vi "File Write.vi"(7 "State Control":enum16{"Open", "Write", "Close"}(ring), 8 "error in (no error)":errorcluster, 10 "Event Data String":string, 11 "Event String":string) -> (0 "error out":errorcluster)   [LabVIEW 2020]
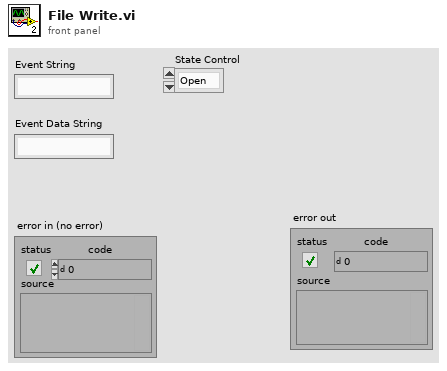
[diagram p1: front panel]
types:
  T1 = enum16{"open", "replace", "create", "open or create", "replace or create", "replace or create with confirmation"}
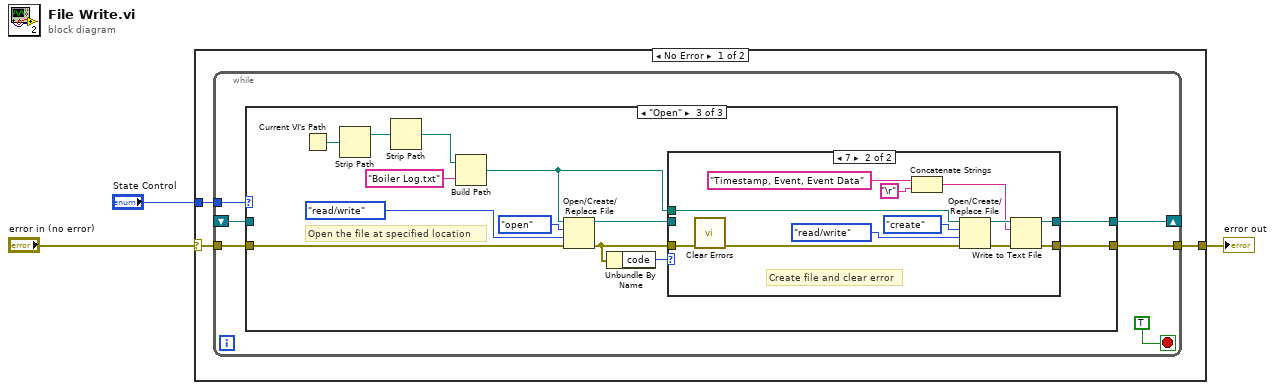
[diagram p0: block diagram]
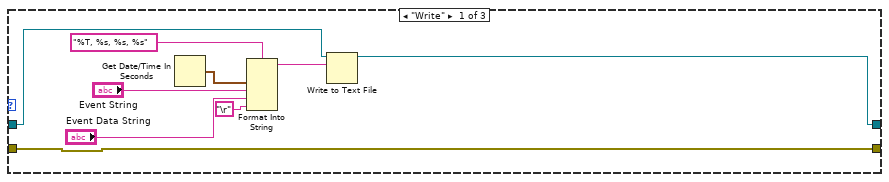
[diagram p2: hidden frame]
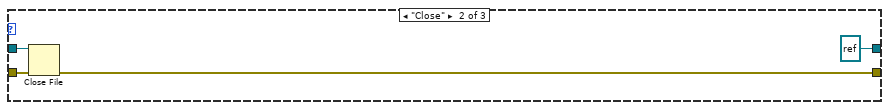
[diagram p3: hidden frame]
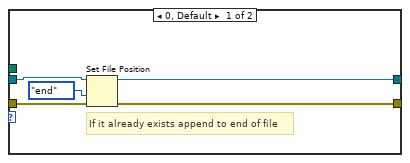
[diagram p4: hidden frame]
diagram:
  n1 = case shown="No Error" "error in (no error)" {
    selector: "error in (no error)" -> [w6 w56]
    tunnel: [w5 w56] -> w1
    tunnel: "State Control" -> [w4 _]
    frame No Error {
      n2 = while {
        tunnel: w4 -> [w10]
        shift-right: [w8] -> _
        shift-left: _ -> [w7]
        tunnel: w6 -> [w12]
        tunnel: [w11] -> w5
        stop <- TRUE stop-if-true
        n3 = case shown="\"Open\"" w10 {
          tunnel: w12 -> [w19 w23 w37]
          tunnel: [w19 w24 w32] -> w11
          tunnel: [w17 refnum<file> refnum ("refnum out") w29] -> w8
          tunnel: w7 -> [w18 w25 _]
          frame "Write" {
            n4 = Get Date/Time In Seconds() -> (seconds since 1Jan1904=w14:timestamp)
            n5 = Format Into String(format string="%T, %s, %s, %s", w14, "Event String", "Event Data String", "\r") -> (resulting string=w16:string)  [unwired: 2 in, 1 out]
            n6 = Write to Text File(file (use dialog)=w18, text=w16) -> (refnum out=w17:refnum<file>)  [unwired: 2 in, 2 out]
          }
          frame "Close" {
            n7 = Close File(refnum=w25, error in=w23) -> (error out=w24:errorcluster)  [unwired: 1 out]
          }
          frame "Open" {
            # "Open the file at specified location"
            n8 = Current VI's Path() -> (path=w38:path)
            n9 = Strip Path(path=w38) -> (stripped path=w35:path)  [unwired: 1 out]
            n10 = Strip Path(path=w35) -> (stripped path=w26:path)  [unwired: 1 out]
            n11 = Build Path(base path=w26, name or relative path="Boiler Log.txt") -> (appended path=w28:path)
            n12 = Open/Create/Replace File(file path (use dialog)=w28, error in=w37, operation (0:open)=T1."open", access (0:read/write)=enum16{"read/write", "read-only", "write-only"}."read/write") -> (refnum out=w30:refnum<file>, error out=w33:errorcluster)  [unwired: 2 in, 1 out]
            n13 = Unbundle By Name(w33) -> ("code"=w34:i32)
            n14 = case shown="7" w34 {
              tunnel: w33 -> [w43 w52]
              tunnel: [w42 w47] -> w32
              tunnel: w30 -> [w41 _]
              tunnel: [w40 w49] -> w29
              tunnel: w28 -> [_ w54]
              frame 0, Default {
                # "If it already exists append to end of file"
                n15 = Set File Position(refnum=w41, from (0:start)=enum16{"start", "end", "current"}."end", error in=w43) -> (refnum out=w40:refnum<file>, error out=w42:errorcluster)  [unwired: 1 in]
              }
              frame 7 {
                # "Create file and clear error"
                n16 = call <vilib>:"Clear Errors.vi"("error in (no error)"=w52) -> ("error out"=w50:errorcluster)  [unwired: 5 in, 1 out]
                n17 = Concatenate Strings("Timestamp, Event, Event Data", "\r") -> (w45:string)
                n18 = Open/Create/Replace File(file path (use dialog)=w54, error in=w50, operation (0:open)=T1."create", access (0:read/write)=enum16{"read/write", "read-only", "write-only"}."read/write") -> (refnum out=w55:refnum<file>, error out=w48:errorcluster)  [unwired: 2 in, 1 out]
                n19 = Write to Text File(file (use dialog)=w55, text=w45, error in=w48) -> (refnum out=w49:refnum<file>, error out=w47:errorcluster)  [unwired: 1 in, 1 out]
              }
            }
          }
        }
      }
    }
    frame Error {
    }
  }
  "error out" <- w1
